vi "InitProgressBar.vi"(8 "error in (no error)":errorcluster, 11 "count":i32) -> (0 "error out":errorcluster, 3 "reference out":refnum<vi>)   [LabVIEW 2017]
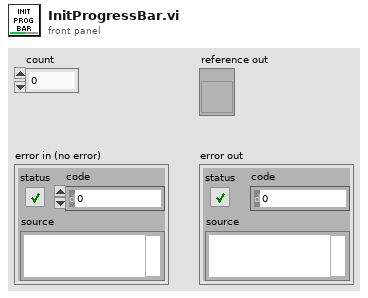
[diagram p1: front panel]
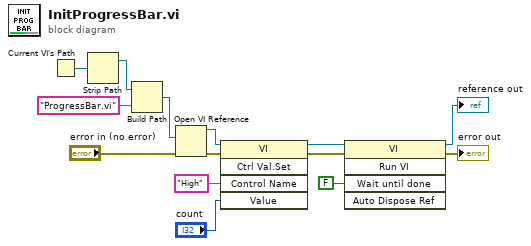
[diagram p0: block diagram]
diagram:
  n1 = Current VI's Path() -> (path=w3:path)
  n2 = Strip Path(path=w3) -> (stripped path=w2:path)  [unwired: 1 out]
  n3 = Build Path(base path=w2, name or relative path="ProgressBar.vi") -> (appended path=w14:path)
  n4 = Open VI Reference(vi path=w14, error in (no error)="error in (no error)") -> (vi reference=w7:refnum<vi>, error out=w6:errorcluster)  [unwired: 4 in]
  n5 = invoke class="VI" method="Ctrl Val.Set"(reference=w7, error in=w6, "Control Name"="High", "Value"="count") -> (reference out=w5:refnum<vi>, error out=w4:errorcluster)  [unwired: 1 in, 3 out]
  n6 = invoke class="VI" method="Run VI"(reference=w5, error in=w4, "Wait until done"=FALSE) -> (reference out=→"reference out":refnum<vi>, error out=→"error out":errorcluster)  [unwired: 2 in, 3 out]
